vi "5_Sychronization.vi"() -> ()   [LabVIEW 2015]
uses:
  C:/Users/MX-Microscope/Documents/LabVIEW Data/lvoop_campus_2018/Detector_Class/Swabian/time_tagger_vis/TTCSharp32.dll
  TTCSharp32.dll
panel:
  out "with Sync":dbl[](array[numeric])
  out "without Sync":dbl[](array[numeric])
  # "The execution of the \"sync\" method ensures that all settings are actually\napplied (in this case the activation of test signal) and the USB buffer is\nflushed. I.e., after a \"sync\" call, we are sure not to receive time tags that\nwere generated in the past. In this demonstration, we turn on the test signal\nand subsequently record the average click rate. One may expect to obtain\nthe original click rate of the test signal. However, data transmission is never\ninstantaneous and therefore we include a time span when the test signal was not\nyet turned on. Consequently, the average click rate is reduced compared to the\nactual value. By inserting a \"sync\" call before we start recording, the\nbehavior is changed and we ensure that we are not processing past time tags.\nTherefore, the average corresponds to the physical click rate."
  # "counts / s"
  # "counts / s"
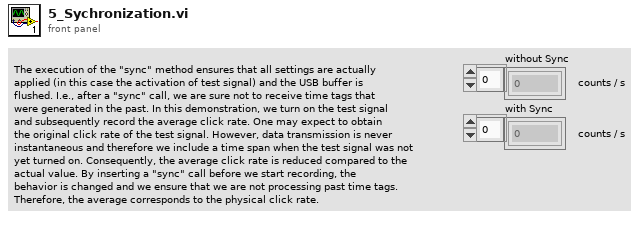
[diagram p1: front panel]
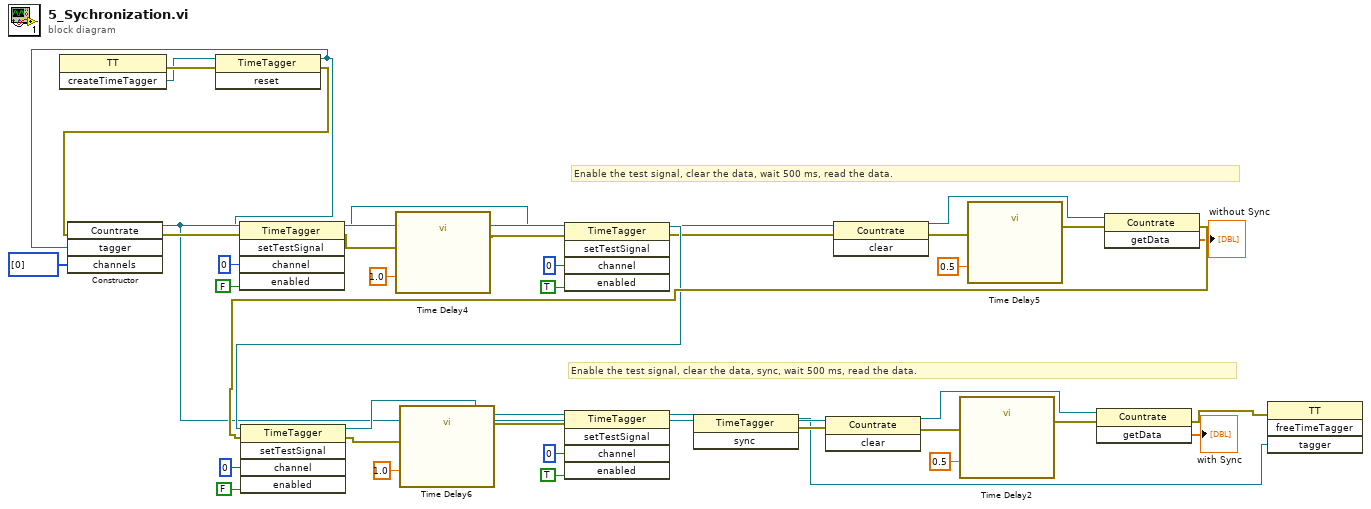
[diagram p0: block diagram]
diagram:
  # "Enable the test signal, clear the data, sync, wait 500 ms, read the data."
  # "Enable the test signal, clear the data, wait 500 ms, read the data."
  n1 = invoke class="TT" method="createTimeTagger"() -> (error out=w40:errorcluster, "createTimeTagger"=w39:refnum<k24>)  [unwired: 3 in, 1 out]
  n2 = invoke class="TimeTagger" method="reset"(reference=w39, error in=w40) -> (reference out=w1:refnum<k24>, error out=w2:errorcluster)  [unwired: 1 in, 1 out]
  n3 = constructor class="Countrate"(error in=w2, "tagger"=w1, "channels"=u32[] [0]) -> (reference out=w10:refnum<k24>, error out=w18:errorcluster)  [unwired: 2 in, 3 out]
  n4 = invoke class="TimeTagger" method="setTestSignal"(reference=w1, error in=w18, "channel"=u32 0, "enabled"=FALSE) -> (reference out=w4:refnum<k24>, error out=w17:errorcluster)  [unwired: 1 in, 3 out]
  n5 = call "Time Delay4"("error in (no error)"=w17, "Delay Time (s)"=1.0) -> ("error out"=w33:errorcluster)  [unwired: 9 in]
  n6 = invoke class="TimeTagger" method="setTestSignal"(reference=w4, error in=w33, "channel"=u32 0, "enabled"=TRUE) -> (reference out=w25:refnum<k24>, error out=w16:errorcluster)  [unwired: 1 in, 3 out]
  n7 = invoke class="Countrate" method="clear"(reference=w10, error in=w16) -> (reference out=w30:refnum<k24>, error out=w32:errorcluster)  [unwired: 1 in, 1 out]
  n8 = call "Time Delay5"("error in (no error)"=w32, "Delay Time (s)"=0.5) -> ("error out"=w29:errorcluster)  [unwired: 9 in]
  n9 = invoke class="Countrate" method="getData"(reference=w30, error in=w29) -> (error out=w26:errorcluster, "getData"=→"without Sync":dbl[])  [unwired: 1 in, 1 out]
  n10 = invoke class="TimeTagger" method="setTestSignal"(reference=w25, error in=w26, "channel"=u32 0, "enabled"=FALSE) -> (reference out=w20:refnum<k24>, error out=w23:errorcluster)  [unwired: 1 in, 3 out]
  n11 = call "Time Delay6"("error in (no error)"=w23, "Delay Time (s)"=1.0) -> ("error out"=w19:errorcluster)  [unwired: 9 in]
  n12 = invoke class="TimeTagger" method="setTestSignal"(reference=w20, error in=w19, "channel"=u32 0, "enabled"=TRUE) -> (reference out=w15:refnum<k24>)  [unwired: 1 in, 4 out]
  n13 = invoke class="TimeTagger" method="sync"(reference=w15) -> (reference out=w5:refnum<k24>, error out=w9:errorcluster)  [unwired: 2 in, 1 out]
  n14 = invoke class="Countrate" method="clear"(reference=w10, error in=w9) -> (reference out=w12:refnum<k24>, error out=w14:errorcluster)  [unwired: 1 in, 1 out]
  n15 = call "Time Delay2"("error in (no error)"=w14, "Delay Time (s)"=0.5) -> ("error out"=w11:errorcluster)  [unwired: 9 in]
  n16 = invoke class="Countrate" method="getData"(reference=w12, error in=w11) -> (error out=w6:errorcluster, "getData"=→"with Sync":dbl[])  [unwired: 1 in, 1 out]
  n17 = invoke class="TT" method="freeTimeTagger"(error in=w6, "tagger"=w5) -> ()  [unwired: 2 in, 4 out]
